vi "Time Out.vi"(11 "Time Out in":T1 {"Time Out Time (s)" format="%#_13g"}) -> (3 "Time Out out":T1 {"Time Out Time (s)" format="%#_13g"})   [LabVIEW 2014]
uses:
  Time Out.ctl
panel:
  out "Elapsed Time (s)":dbl
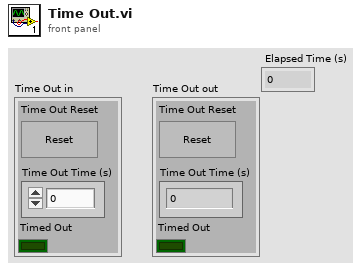
[diagram p1: front panel]
types:
  T1 = typedef "Time Out.ctl" = cluster{"Time Out Reset":bool, "Timed Out":bool, "Time Out Time (s)":dbl}
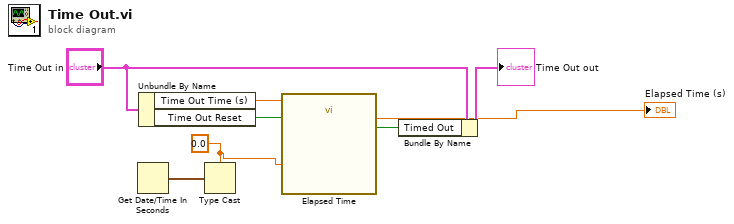
[diagram p0: block diagram]
diagram:
  w1 = 0.0 ("type")
  n1 = Get Date/Time In Seconds() -> (seconds since 1Jan1904=w3:timestamp)
  n2 = Unbundle By Name("Time Out in") -> ("Time Out Time (s)"=w4:dbl, "Time Out Reset"=w5:bool)
  n3 = Type Cast(type=w1, x=w3) -> ()  [unwired: 1 out]
  n4 = call "Elapsed Time"("Time Target (s)"=w4, "Reset"=w5, "Set Start Time (s)"=w1) -> ("Elapsed Time (s)"=→"Elapsed Time (s)":dbl, "Time has Elapsed"=w7:bool)  [unwired: 9 in, 6 out]
  n5 = Bundle By Name(cluster="Time Out in", "Timed Out"=w7) -> (→"Time Out out":T1)
